vi "Modbus Async.vi"(10 "Parameters":variant, 11 "Process":refnum<class "Process.lvclass">) -> ()   [LabVIEW 2020, in "Modbus Master Engine.lvlib"]
uses:
  Modbus Master Engine.lvlib
  <vilib>/NI/NIVS Inline Async API/_VS Inline Async API/Process/Process.lvclass
  Custom Device/Shared/Device Info.ctl
  Custom Device/Shared/Write Mode.ctl
  Custom Device/Shared/Controls/Interface Type.ctl
  Custom Device/Shared/Controls/Data Model/TCP Settings.ctl
  Custom Device/Shared/Controls/Data Model/Serial Settings.ctl
  Custom Device/Shared/Bulk Data Access.ctl
  Custom Device/System Explorer/SubVIs/Modbus Type.ctl
  Custom Device/Shared/Controls/Data Model/Channel.ctl
  <vilib>/NI VeriStand/Custom Device API/Custom Device Channel Type.ctl
  Custom Device/Shared/Controls/Data Model/Mapping.ctl
  Custom Device/Shared/Controls/Data Model/DataType.ctl
  <vilib>/NI VeriStand/Custom Device API/Custom Device Item Ref.ctl
  <vilib>/NI/NIVS Inline Async API/_VS Inline Async API/Process/Process.lvclass/Process.ctl
  API/Slave/Modbus Slave.lvclass
  C:/Users/Administrator/Desktop/GIT/Modbus-Custom-Device-v2/Source/Custom Device Support/API/Modbus API.lvclass
  API/Master/Modbus Master.lvclass
  <vilib>/NI/NIVS Inline Async API/_VS Inline Async API/Error Handling Process/SubVIs/Error.ConvertArray.vi
  API/Modbus API.lvclass
  Custom Device/Shared/Modbus Master Shared.lvlib
  <vilib>/NI VeriStand/Custom Device API/Custom Device API.lvlib
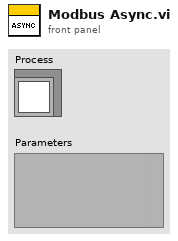
[diagram p1: front panel]
types:
  T1 = typedef "Modbus Master Shared.lvlib/Device Info.ctl" = cluster{"Interface Data":cluster{"Name":string, "Unit ID":u8, "Refresh Rate":i32, "Write Rate":i32, "Write Mode":T2, "Interface Type":T3, "TCP Settings":T4, "Serial Settings":T5}, "Modbus Input Groups":T6[], "Modbus Output Groups":T6[], "error in (no error)":errorcluster, "Modbus Input Engine Group Names":string[], "Modbus Output Engine Group Names":string[]}
  T2 = typedef "Modbus Master Shared.lvlib/Write Mode.ctl" = enum16{"Value Change", "Interval"}
  T3 = typedef "Modbus Master Shared.lvlib/Interface Type.ctl" = enum16{"TCP Master", "Serial Master", "TCP Slave", "Serial Slave"}
  T4 = typedef "Modbus Master Shared.lvlib/TCP Settings.ctl" = cluster{"Address":string, "Port":u16, "Timeout":i32}
  T5 = typedef "Modbus Master Shared.lvlib/Serial Settings.ctl" = cluster{"VISA resource name":refnum<visa-resource-name>, "baud rate":u32, "parity (even)":u16, "flow control (none)":u16, "serial type":enum16{"RTU", "ASCII"}, "Wire Mode":i16}
  T6 = typedef "Modbus Master Shared.lvlib/Bulk Data Access.ctl" = cluster{"Modbus Type":T7, "start":u16, "length":u16, "Channel Data":T8[]}
  T7 = typedef "Modbus Master Shared.lvlib/Modbus Type.ctl" = enum16{"Coil", "Discrete Input", "Holding Register", "Input Register"}
  T8 = typedef "Modbus Master Shared.lvlib/Channel.ctl" = cluster{"Name":string, "Modbus Type":T7, "Veristand Type":T9, "Mapping":T10}
  T9 = typedef "Custom Device API.lvlib/Custom Device Channel Type.ctl" = enum16{"Input", "Output"}
  T10 = typedef "Modbus Master Shared.lvlib/Mapping.ctl" = cluster{"DataType":T11, "Starting Address":u16, "Sub-Index (Bool)":u16, "VS Reference":T12}
  T11 = typedef "Modbus Master Shared.lvlib/DataType.ctl" = enum16{"Double", "Single", "I64", "I32", "I16", "I8", "U64", "U32", "U16", "U8", "Boolean"}
  T12 = typedef "Custom Device API.lvlib/Custom Device Item Ref.ctl" = u64
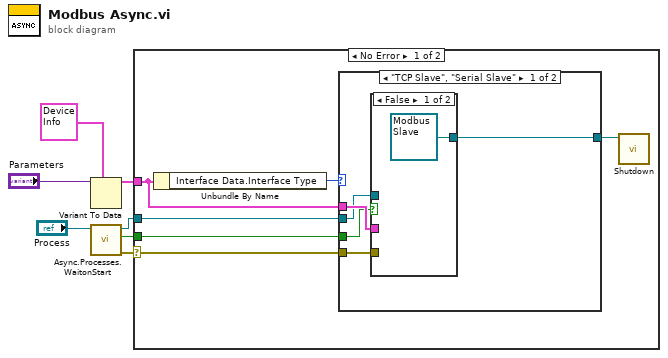
[diagram p0: block diagram]
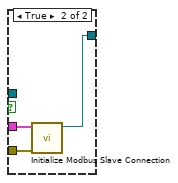
[diagram p2: hidden frame]
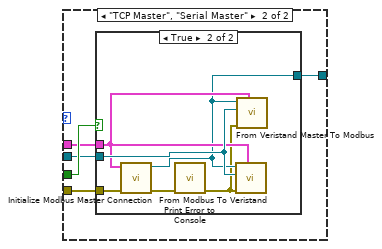
[diagram p3: hidden frame]
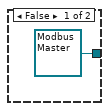
[diagram p4: hidden frame]
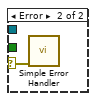
[diagram p5: hidden frame]
diagram:
  n1 = Variant To Data(type=T1 {"Interface Data"={"Name"="", "Unit ID"=0, "Refresh Rate"=0, "Write Rate"=0, "Write Mode"=enum."Value Change", "Interface Type"=enum."TCP Master", "TCP Settings"={"Address"="", "Port"=0, "Timeout"=0}, "Serial Settings"={"VISA resource name"="", "baud rate"=0, "parity (even)"=0, "flow control (none)"=0, "serial type"=enum."RTU", "Wire Mode"=-1}}, "Modbus Input Groups"=[], "Modbus Output Groups"=[], "error in (no error)"={"status"=FALSE, "code"=0, "source"=""}, "Modbus Input Engine Group Names"=[], "Modbus Output Engine Group Names"=[]} ("Parameters"), Variant="Parameters") -> (data=w1:T1)  [unwired: 1 in, 1 out]
  n2 = call <vilib>:"Async.Processes.WaitonStart.vi"("Process"="Process") -> ("error out"=w5:errorcluster, "Execute"=w6:bool, "Process out"=w4:refnum<class "Process.lvclass">)  [unwired: 8 in]
  n3 = case shown="No Error" w5 {
    selector: w5 -> [w12 w35]
    tunnel: w1 -> [w10 _]
    tunnel: w6 -> [w13 _]
    tunnel: w4 -> [w11 _]
    frame No Error {
      n4 = Unbundle By Name(w10) -> ("Interface Data.Interface Type"=w9:T3)
      n5 = case shown="\"TCP Slave\", \"Serial Slave\"" w9 {
        tunnel: w13 -> [w14 w27]
        tunnel: w12 -> [w18 w26]
        tunnel: w11 -> [w16 w25]
        tunnel: w10 -> [w17 w24]
        tunnel: [w15 w23] -> w8
        frame "TCP Slave", "Serial Slave" {
          n6 = case shown="False" w14 {
            tunnel: w18 -> [_ w22]
            tunnel: w17 -> [_ w21]
            tunnel: w16 -> [_ _]
            tunnel: [refnum<class "Modbus Slave.lvclass"> refnum ("Modbus Slave Out") w20] -> w15
            frame False {
            }
            frame True {
              n7 = call "Initialize Modbus Slave Connection.vi"("error in (no error)"=w22, "Parameters"=w21) -> ("Modbus Slave Out"=w20:refnum<class "Modbus Slave.lvclass">)  [unwired: 8 in, 1 out]
            }
          }
        }
        frame "TCP Master", "Serial Master" {
          n8 = case shown="True" w27 {
            tunnel: w26 -> [_ w34]
            tunnel: w24 -> [_ w32]
            tunnel: w25 -> [_ w33]
            tunnel: [refnum<class "Modbus Master.lvclass"> refnum ("Modbus Master out") w31] -> w23
            frame False {
            }
            frame True {
              n9 = call "Initialize Modbus Master Connection.vi"("error in (no error)"=w34, "Parameters"=w32) -> ("error out"=w30:errorcluster, "Modbus Master out"=w31:refnum<class "Modbus Master.lvclass">)  [unwired: 8 in]
              n10 = call "Print Error to Console.vi"("error in (no error)"=w30) -> ("error out"=w29:errorcluster)  [unwired: 10 in]
              n11 = call "From Modbus To Veristand.vi"("Parameters"=w32, "error in (no error)"=w29, "Process in"=w33, "Modbus API.lvlibp:Modbus Master"=w31) -> ()  [unwired: 8 in]
              n12 = call "From Veristand Master To Modbus.vi"("Parameters"=w32, "error in (no error)"=w29, "Process in"=w33, "Modbus Master in"=w31) -> ()  [unwired: 8 in]
            }
          }
        }
      }
      n13 = call-dynamic "Shutdown.vi"("Modbus instance in"=w8) -> ()  [unwired: 10 in, 1 out]
    }
    frame Error {
      n14 = call <vilib>:"Simple Error Handler.vi"("error in (no error)"=w35) -> ()  [unwired: 4 in, 5 out]
    }
  }
